vi "Query Sequencer ARB File Pool Valid.vi"(8 "error in (no error)":errorcluster, 10 "Instance (1)":i32=1, 11 "VISA resource name":refnum<visa-resource-name>) -> (0 "error out":errorcluster, 2 "Valid":i32, 3 "VISA resource name out":refnum<visa-resource-name>)   [LabVIEW 2020, in "Rohde&Schwarz CMXP GPRF.lvlib"]
doc: "Queries whether the ARB file pool is valid.\n\nAttribute:\nRSCMXPGPRF_ATTR_SEQUENCER_ARB_FILE_POOL_VALID\n\nRemote-control command:\nSOURce:GPRF:GEN<i>:SEQuencer:APOol:VALid?"
uses:
  <instrlib>/Rohde&Schwarz CMXP GPRF/Rohde&Schwarz CMXP GPRF.lvlib
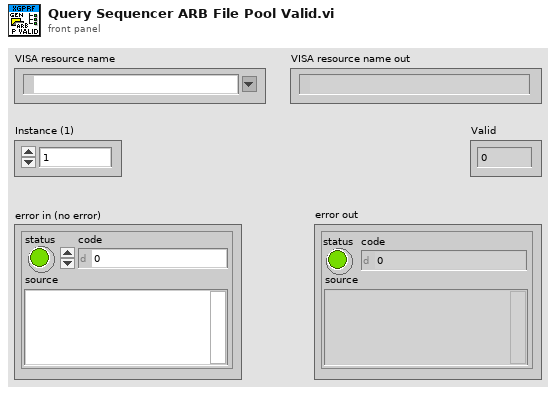
[diagram p1: front panel]
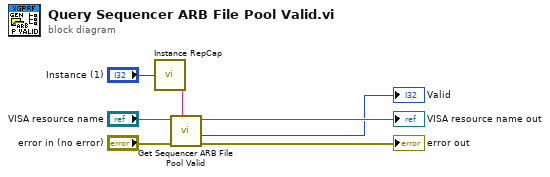
[diagram p0: block diagram]
diagram:
  n1 = call <instrlib>:"Instance RepCap.vi"("Instance in"="Instance (1)") -> ("Instance out"=w2:string)
  n2 = call "Get Sequencer ARB File Pool Valid"("Repeated Capabilities"=w2, "error in (no error)"="error in (no error)", "instrument handle"="VISA resource name") -> ("error out"=→"error out":errorcluster, "Sequencer ARB File Pool Valid"=→"Valid":i32, "instrument handle out"=→"VISA resource name out":refnum<visa-resource-name>)  [unwired: 6 in]
